vi "Plot My Scheduler Result.vi"(7 "Fitness Value":i32, 8 "error in (no error)":errorcluster, 9 "Number of Jobs":i32, 10 "Number of Machines":i32, 11 "Gannt Chart In":T1[][](array[typedef])) -> (0 "error out":errorcluster, 3 "My Scheduler Graph":picture)   [LabVIEW 2013, in "Scheduler.lvclass"]
uses:
  Scheduler.lvclass
  Controls/GanntChart_Element.ctl
  <vilib>/Heliosphere Research LLC/Advanced Plotting Toolkit/typedefs/PlotColor.ctl
  <vilib>/Heliosphere Research LLC/Advanced Plotting Toolkit/api_figure/TicksProperties.ctl
  <vilib>/Heliosphere Research LLC/Advanced Plotting Toolkit/properties/Text.ctl
  <vilib>/Heliosphere Research LLC/Advanced Plotting Toolkit/properties/Text_FontSize.ctl
  <vilib>/Heliosphere Research LLC/Advanced Plotting Toolkit/properties/Text_FontStyle.ctl
  <vilib>/Heliosphere Research LLC/Advanced Plotting Toolkit/api_annotations/ShapeProperties.ctl
  <vilib>/Heliosphere Research LLC/Advanced Plotting Toolkit/properties/Line.ctl
  <vilib>/Heliosphere Research LLC/Advanced Plotting Toolkit/properties/Line_Style.ctl
  <vilib>/Heliosphere Research LLC/Advanced Plotting Toolkit/properties/Display.ctl
  <vilib>/Heliosphere Research LLC/Advanced Plotting Toolkit/api_annotations/TextProperties.ctl
  <vilib>/Heliosphere Research LLC/Advanced Plotting Toolkit/Advanced Plotting Toolkit.lvlib
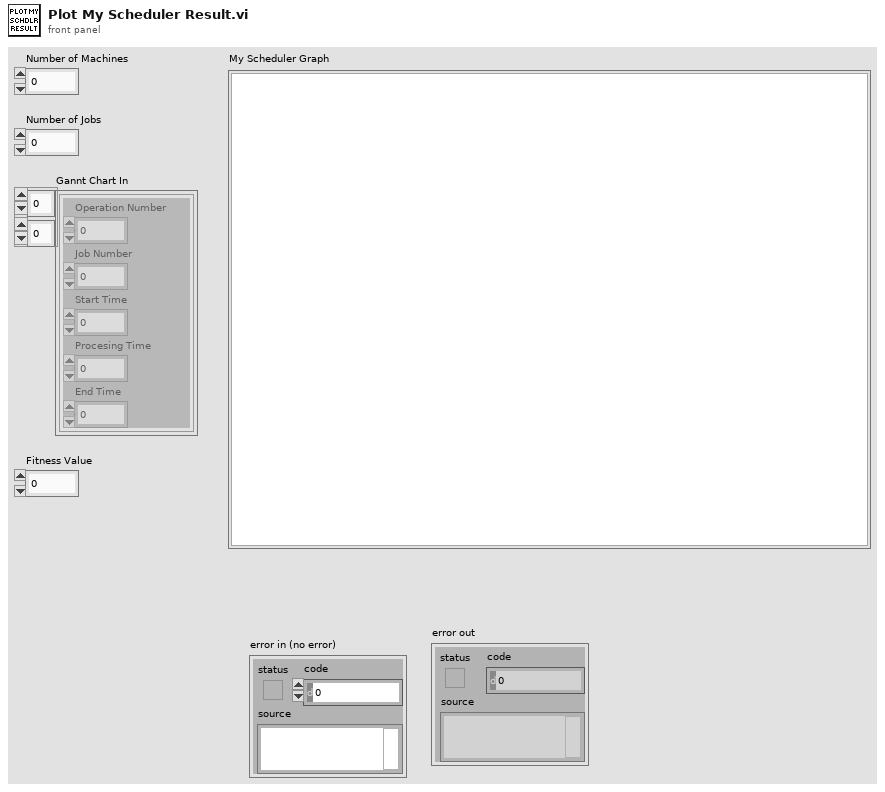
[diagram p1: front panel]
types:
  T1 = typedef "GanntChart_Element.ctl" = cluster{"Operation Number":i32, "Job Number":i32, "Start Time":i32, "Procesing Time":u16, "End Time":i32}
  T2 = typedef "Advanced Plotting Toolkit.lvlib/Text_FontSize.ctl" = i32
  T3 = typedef "Advanced Plotting Toolkit.lvlib/TicksProperties.ctl" = cluster{"Text":T4}
  T4 = typedef "Advanced Plotting Toolkit.lvlib/Text.ctl" = cluster{"Color":T5, "Background Color":T5, "Font Size (points)":T2, "Font Style":T6, "Rotation Angle":dbl}
  T5 = typedef "Advanced Plotting Toolkit.lvlib/PlotColor.ctl" = u32
  T6 = typedef "Advanced Plotting Toolkit.lvlib/Text_FontStyle.ctl" = enum16{"Automatic", "Normal", "Italic", "Bold"}
  T7 = typedef "Advanced Plotting Toolkit.lvlib/PlotID.ctl" = i32
  T8 = typedef "Advanced Plotting Toolkit.lvlib/TextProperties.ctl" = cluster{"Text":T4, "Display":T9}
  T9 = typedef "Advanced Plotting Toolkit.lvlib/Display.ctl" = cluster{"Alpha":dbl, "Z Order":dbl}
  T10 = typedef "Advanced Plotting Toolkit.lvlib/ShapeProperties.ctl" = cluster{"Color":T5, "Line":T11, "Display":T9}
  T11 = typedef "Advanced Plotting Toolkit.lvlib/Line.ctl" = cluster{"Style":T12, "Color":T5, "Width":sgl}
  T12 = typedef "Advanced Plotting Toolkit.lvlib/Line_Style.ctl" = enum16{"Automatic", "Solid", "Dashed", "Dotted", "Dash-dot", "Invisible"}
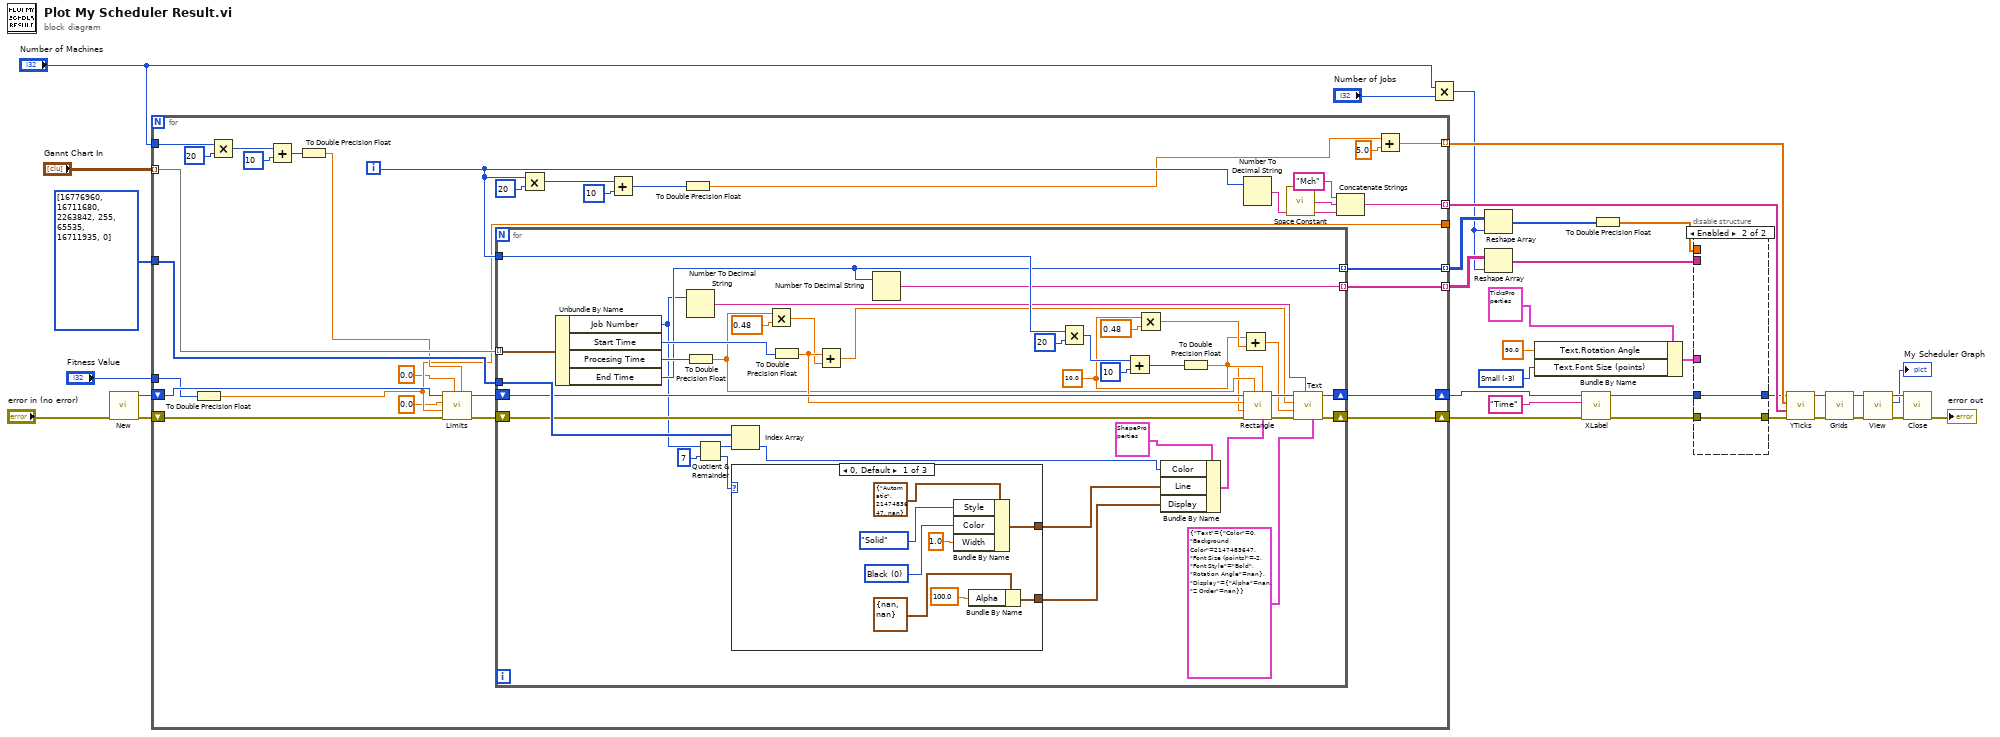
[diagram p0: block diagram]
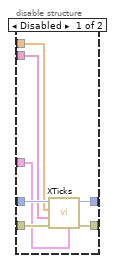
[diagram p2: hidden frame]
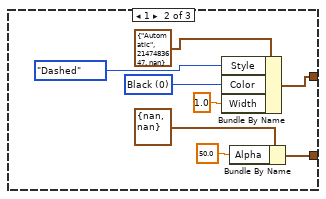
[diagram p3: hidden frame]
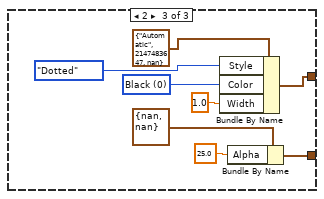
[diagram p4: hidden frame]
diagram:
  w8 = T2 -3 items=["Automatic"=0, "XX-Small"=-1, "X-Small"=-2, "Small"=-3, "Medium"=-4, "Large"=-5, "X-Large"=-6, "XX-Large"=-7] ("Text.Font Size (points)")
  w29 = T5[] [16776960, 16711680, 2263842, 255, 65535, 16711935, 0] items=["Automatic"=2147483647, "Black"=0, "White"=16777215, "Red"=16711680, "Green"=2263842, "Blue"=255, "Cyan"=65535, "Magenta"=16711935, "Yellow"=16776960]
  n1 = call <vilib>:"New.vi"("error in (no error)"="error in (no error)") -> ("error out"=w30:errorcluster, "Plot ID"=w31:T7)  [unwired: 9 in]
  n2 = for {
    shift-right: [w67] -> w27
    shift-left: w30 -> [w63]
    shift-right: [w66] -> w28
    shift-left: w31 -> [w61]
    tunnel: "Gannt Chart In" -> [w65] mode=indexing
    tunnel: w29 -> [w64]
    tunnel: [w53] -> w21 mode=indexing
    tunnel: [w43] -> w20 mode=indexing
    tunnel: [w42] -> w7 mode=indexing
    tunnel: [w41] -> w15 mode=indexing
    tunnel: [w40] -> _
    tunnel: "Number of Machines" -> [w39]
    tunnel: "Fitness Value" -> [w38]
    i -> [w46]
    n3 = To Double Precision Float(number=w38) -> (double precision float=w40:dbl)
    n4 = Multiply(x=w39, y=20) -> (x*y=w59:i32)
    n5 = Add(x=w59, y=10) -> (x+y=w57:i32)
    n6 = To Double Precision Float(number=w57) -> (double precision float=w51:dbl)
    n7 = call <vilib>:"Limits.vi"("Y Max"=w51, "Y Min"=0.0, "error in (no error)"=w63, "X Max"=w40, "X Min"=0.0, "Plot ID"=w61) -> ("error out"=w62:errorcluster, "Plot ID Out"=w56:T7)  [unwired: 4 in]
    n8 = for {
      shift-right: [w81] -> w67
      shift-left: w62 -> [w103]
      shift-right: [w83] -> w66
      shift-left: w56 -> [w102]
      tunnel: w65 -> [w105] mode=indexing
      tunnel: w64 -> [w104]
      tunnel: w46 -> [w92]
      tunnel: [w86] -> w42 mode=indexing
      tunnel: [w85] -> w41 mode=indexing
      w73 = 10.0 ("Height")
      n9 = Unbundle By Name(w105) -> ("Job Number"=w70:i32, "Start Time"=w97:i32, "Procesing Time"=w98:u16, "End Time"=w86:i32)
      n10 = Number To Decimal String(number=w70) -> (decimal integer string=w69:string)  [unwired: 1 in]
      n11 = To Double Precision Float(number=w98) -> (double precision float=w79:dbl)
      n12 = Quotient & Remainder(x=w70, y=7) -> (x-y*floor(x/y)=w89:i32, floor(x/y)=w88:i32)
      n13 = Index Array(array=w104, index=w89) -> (element=w99:T5)
      n14 = case shown="0, Default" w88 {
        tunnel: [w109 w117 w125] -> w91
        tunnel: [w106 w114 w122] -> w87
        frame 0, Default {
          w111 = T5 0 items=["Automatic"=2147483647, "Black"=0, "White"=16777215, "Red"=16711680, "Green"=2263842, "Blue"=255, "Cyan"=65535, "Magenta"=16711935, "Yellow"=16776960] ("Color")
          n15 = Bundle By Name(cluster=T11 {"Style"=enum."Automatic", "Color"=2147483647, "Width"=nan} ("Line"), "Style"=Line_Style."Solid", "Color"=w111, "Width"=sgl 1.0) -> (w109:T11)
          n16 = Bundle By Name(cluster=T9 {"Alpha"=nan, "Z Order"=nan} ("Display"), "Alpha"=100.0) -> (w106:T9)
        }
        frame 1 {
          w119 = T5 0 items=["Automatic"=2147483647, "Black"=0, "White"=16777215, "Red"=16711680, "Green"=2263842, "Blue"=255, "Cyan"=65535, "Magenta"=16711935, "Yellow"=16776960] ("Color")
          n17 = Bundle By Name(cluster=T11 {"Style"=enum."Automatic", "Color"=2147483647, "Width"=nan} ("Line"), "Style"=Line_Style."Dashed", "Color"=w119, "Width"=sgl 1.0) -> (w117:T11)
          n18 = Bundle By Name(cluster=T9 {"Alpha"=nan, "Z Order"=nan} ("Display"), "Alpha"=50.0) -> (w114:T9)
        }
        frame 2 {
          w127 = T5 0 items=["Automatic"=2147483647, "Black"=0, "White"=16777215, "Red"=16711680, "Green"=2263842, "Blue"=255, "Cyan"=65535, "Magenta"=16711935, "Yellow"=16776960] ("Color")
          n19 = Bundle By Name(cluster=T11 {"Style"=enum."Automatic", "Color"=2147483647, "Width"=nan} ("Line"), "Style"=Line_Style."Dotted", "Color"=w127, "Width"=sgl 1.0) -> (w125:T11)
          n20 = Bundle By Name(cluster=T9 {"Alpha"=nan, "Z Order"=nan} ("Display"), "Alpha"=25.0) -> (w122:T9)
        }
      }
      n21 = Multiply(x=w79, y=0.48) -> (x*y=w77:dbl)
      n22 = To Double Precision Float(number=w97) -> (double precision float=w80:dbl)
      n23 = Add(x=w80, y=w77) -> (x+y=w76:dbl)
      n24 = Number To Decimal String(number=w86) -> (decimal integer string=w85:string)  [unwired: 1 in]
      n25 = Multiply(x=w92, y=20) -> (x*y=w95:i32)
      n26 = Add(x=w95, y=10) -> (x+y=w93:i32)
      n27 = Multiply(x=w73, y=0.48) -> (x*y=w75:dbl)
      n28 = Bundle By Name(cluster=T10 {"Color"=2147483647, "Line"={"Style"=enum."Automatic", "Color"=2147483647, "Width"=nan}, "Display"={"Alpha"=nan, "Z Order"=nan}} ("Properties"), "Color"=w99, "Line"=w91, "Display"=w87) -> (w100:T10)
      n29 = To Double Precision Float(number=w93) -> (double precision float=w72:dbl)
      n30 = Add(x=w72, y=w75) -> (x+y=w71:dbl)
      n31 = call <vilib>:"Rectangle.vi"("Properties"=w100, "Height"=w73, "Width"=w79, "error in (no error)"=w103, "Y Position"=w72, "X Position"=w80, "Plot ID"=w102) -> ("error out"=w82:errorcluster, "Plot ID Out"=w84:T7)  [unwired: 3 in]
      n32 = call <vilib>:"Text.vi"("Properties"=T8 {"Text"={"Color"=0, "Background Color"=2147483647, "Font Size (points)"=-2, "Font Style"=enum."Bold", "Rotation Angle"=nan}, "Display"={"Alpha"=nan, "Z Order"=nan}}, "Text"=w69, "error in (no error)"=w82, "Y Position"=w71, "X Position"=w76, "Plot ID"=w84) -> ("error out"=w81:errorcluster, "Plot ID Out"=w83:T7)  [unwired: 4 in]
    }
    n33 = Multiply(x=w46, y=20) -> (x*y=w49:i32)
    n34 = Add(x=w49, y=10) -> (x+y=w47:i32)
    n35 = To Double Precision Float(number=w47) -> (double precision float=w45:dbl)
    n36 = Number To Decimal String(number=w46) -> (decimal integer string=w52:string)  [unwired: 1 in]
    n37 = call <vilib>:"Space Constant.vi"() -> ("String"=w54:string)
    n38 = Concatenate Strings("Mch", w54, w52) -> (w53:string)
    n39 = Add(x=w45, y=5.0) -> (x+y=w43:dbl)
  }
  n40 = Multiply(x="Number of Machines", y="Number of Jobs") -> (x*y=w4:i32)
  n41 = Reshape Array(w7, w4) -> (w13:i32[])
  n42 = Reshape Array(w15, w4) -> (w14:string[])
  n43 = Bundle By Name(cluster=T3 {"Text"={"Color"=2147483647, "Background Color"=2147483647, "Font Size (points)"=0, "Font Style"=enum."Automatic", "Rotation Angle"=nan}} ("Properties"), "Text.Rotation Angle"=90.0, "Text.Font Size (points)"=w8) -> (w9:T3)
  n44 = call <vilib>:"XLabel.vi"("error in (no error)"=w27, "Label"="Time", "Plot ID"=w28) -> ("error out"=w17:errorcluster, "Plot ID out"=w19:T7)  [unwired: 7 in]
  n45 = To Double Precision Float(number=w13) -> (double precision float=w12:dbl[])
  n46 = disable-structure shown="Enabled" {
    disable-tunnel: w19 -> [w136 w138]
    disable-tunnel: [w135 w138] -> w18
    disable-tunnel: w17 -> [w134 w137]
    disable-tunnel: [w133 w137] -> w16
    disable-tunnel: w14 -> [w132 _]
    disable-tunnel: w12 -> [w131 _]
    disable-tunnel: w9 -> [w130 _]
    frame Disabled {
      n47 = call <vilib>:"XTicks.vi"("Properties"=w130, "error in (no error)"=w134, "Tick Labels"=w132, "Tick Locations"=w131, "Plot ID"=w136) -> ("error out"=w133:errorcluster, "Plot ID Out"=w135:T7)  [unwired: 5 in]
    }
    frame Enabled {
    }
  }
  n48 = call <vilib>:"YTicks.vi"("error in (no error)"=w16, "Tick Labels"=w21, "Tick Locations"=w20, "Plot ID"=w18) -> ("error out"=w23:errorcluster, "Plot ID Out"=w22:T7)  [unwired: 6 in]
  n49 = call <vilib>:"Grids.vi"("error in (no error)"=w23, "Plot ID"=w22) -> ("error out"=w26:errorcluster, "Plot ID Out"=w24:T7)  [unwired: 8 in]
  n50 = call <vilib>:"View.vi"("error in (no error)"=w26, "Plot ID"=w24) -> ("error out"=w5:errorcluster, "Picture"=→"My Scheduler Graph":picture, "Plot ID Out"=w6:T7)  [unwired: 7 in]
  n51 = call <vilib>:"Close.vi"("error in (no error)"=w5, "Plot ID"=w6) -> ("error out"=→"error out":errorcluster)  [unwired: 9 in]
